vi "DFConfig Save My.Datafinder.vi"(8 "error in (no error)":errorcluster, 10 "my.datafinder (\"\")":string, 11 "my.datafinder Path (empty)":path) -> (0 "error out":errorcluster)   [LabVIEW 2011]
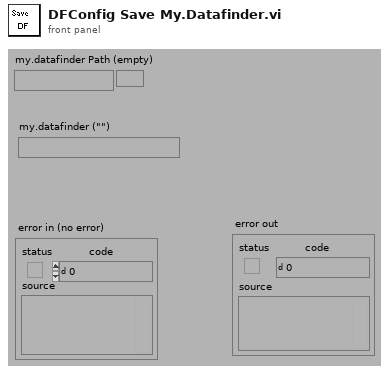
[diagram p1: front panel]
types:
  T1 = enum16{"open", "replace", "create", "open or create", "replace or create", "replace or create with confirmation"}
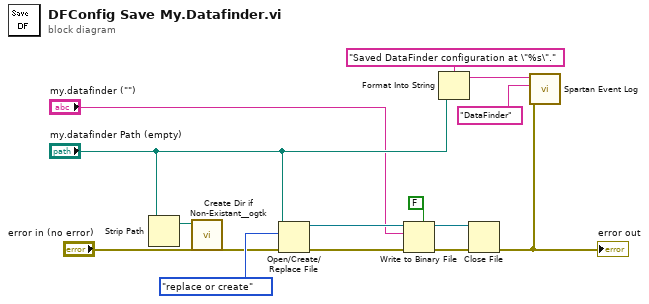
[diagram p0: block diagram]
diagram:
  n1 = Strip Path(path="my.datafinder Path (empty)") -> (stripped path=w10:path)  [unwired: 1 out]
  n2 = call "Create Dir if Non-Existant__ogtk.vi"("error in (no error)"="error in (no error)", "Directory Path"=w10) -> ("error out"=w9:errorcluster)  [unwired: 1 in, 8 out]
  n3 = Open/Create/Replace File(file path (use dialog)="my.datafinder Path (empty)", error in=w9, operation (0:open)=T1."replace or create") -> (refnum out=w11:refnum<file>, error out=w12:errorcluster)  [unwired: 4 out]
  n4 = Write to Binary File(file (use dialog)=w11, data="my.datafinder (\"\")", error in=w12, 5:FALSE) -> (refnum out=w15:refnum<file>, error out=w14:errorcluster)  [unwired: 3 out]
  n5 = Format Into String(format string="Saved DataFinder configuration at \"%s\".", "my.datafinder Path (empty)") -> (resulting string=w3:string)  [unwired: 2 in, 1 out]
  n6 = Close File(refnum=w15, error in=w14) -> (error out=w2:errorcluster)  [unwired: 1 out]
  "error out" <- w2
  n7 = call "Spartan Event Log.vi"("error in (no error)"=w2, "module (\"\")"="DataFinder" ("module (\"\")"), "message (\"\")"=w3) -> ()  [unwired: 2 in, 4 out]
